vi "RSA306 hkplaying2.vi"() -> ()   [LabVIEW 2016]
doc: "This VI demonstrates a simple procedure for setting up a spectrum analyzer, running an acquisition, and retrieving and plotting the waveform data.\n\nString indicators Binary WF Data and Sgl Float WF Data are initialized to empty strings. Waveform Graph is initialized to 0 for 100000 locations (just an arbitrary number for demonstration purposes).\n\ntkrsa6100 Initialize.vi opens the VISA Resource Name from the information entered by the user. It also presets the instrument by default to the Spectrum measurement. On completion it passes dup VISA Resource Name and error out to the following drivers.\n\nThe next VI to execute is tkrsa6100 Config Frequency.vi. Numeric control Center Freq (MHz)(50) is passed to the VI to set the center frequency to the default 50MHz value. The Set/Read Freq Setting (Set) is not wired since it defaults to SET, which is what is desired in this case. This is the case for all the configuration VI's in the example.\n\nThe next VI to execute is tkrsa6100 Config Spectrum Settings.vi. Enumerated control Spectrum Settings (CENTER FREQUENCY) is passed a Frequency Span constant and numeric control Freq Span (MHz) (40) to set the span to 40MHz.\n\nNext the reference level is set using tkrsa6100 Config RF Input.vi. Enumerated control Input Setting (REFERENCE LEVEL) is passed a Reference Level constant and numeric control Ref Level (dBm)(0) to set the reference level to 0dBm.\n\nNext the acquisition mode is set to single acquisition using tkrsa6100 Config Acquisition.vi. No parameters are passed since the default setting of this VI sets the acquisition mode to single.\n\nA single acquisition is then performed using tkrsa6100 Run Single Acquisition.vi. This VI sends an INIT command followed by a *OPC? Query. When the acquisition is completed the instrument returns a 1 and the next vi executes.\n\nThe binary waveform data is then retrieved by tkrsa6100 Spectrum Msmt Results.vi. The last acquisition data is retrieved by passing constant GET LAST ACQUISITION RESULT to enumerated input Run Acquisition and/or Get Result (RUN ACQUISITION & GET RESULT). The binary data is converted to a comma separated list of single precision floating point numbers by passing constant YES to enumerated input Convert Resp String (NO). The number of display points (total number of data bytes/4) is passed to a Spectral Display property node to scale the x axis of the graph. The binary data string from output Measurement Response String is copied to string indicator Binary WF Data. The converted binary data from output Converted Sgl Float Response String is copied to string indicator Sgl Float WF Data.\n\nSgl Float WF Data is then converted to an array by function Spreadsheet String to Array using a comma as the data separator. The output array is then passed to waveform graph Spectral Display for viewing.\n\nThe VISA Resource Name is closed using tkrsa6100 Close.vi."
panel:
  out "Time to Sample":dbl
  out "Total # of Samples":i32
  in  "Freq Out Cluster":T1={"Start Freq (MHz)"=0.0, "Stop Freq (MHz)"=40.0, "Freq Center"=20000000.0, "Freq Step (KHz)"=49.93757802746566, "Acquisition Time (ms)"=0.2181818181818, "Acquisition Samples"=12218.0, "Time Step (sec)"=1.785740859238828e-08, "Spectrum Length"=0.0234894285714, "Spectrum Offset"=-0.0117447142857}
  in  "Freq Center":dbl
  in  "RSA Control Cluster":T2={"Center Freq (MHz)"=20.0, "Freq Span (MHz)"=40.0, "Ref Level (dBm)"=0.0, "# Points"=enum."801", "Analysis Length (ms)"=0.2, "Trigger Settings\n(TRIGGER SOURCE)"=enum."TRIGGER ON"} {"Analysis Length (ms)" step=1e-09; "Ref Level (dBm)" min=-170.0 max=50.0 step=0.1}
  out "cursor diff":dbl
  out "iteration":i32
  out "# of Pts Between Cursors":dbl
  out "Cursor 1 X":dbl
  out "Cursor 0 X":dbl
  in  "I & Q full":cluster{dbl[], "I or Q Data Array":sgl[]}[](graph)=[{array[11200 elements], "I or Q Data Array"=array[11200 elements]}, {array[11200 elements], "I or Q Data Array"=array[11200 elements]}]
  in  "stop":bool
  in  "beta":dbl format="%0.2f"
  in  "Use windowing":bool
  out "FFT^2 from I&Q":cluster{dbl[], dbl[]}[](graph)
  out "FreqStep":dbl
  out "I & Q  partial":cluster{dbl[], sgl[]}[](graph)
  # "This VI has the setup parameters entered in a sub VI\nThe FFT calculation is done in a loop that allows the # of pts\nto FFT to be selected. Also windowing can be changed.\nWhen happy about the FFT then push the STOP button.\nVersion just h is this VI before the setup sub VI was used.\n4/21/17 Version hj moved the memory full causing for loop out of the \nwhile loop. Also added Trigger source to RSA cluster, so it could be\nset to Trigger Off to allow run without pulseblaster trigger."
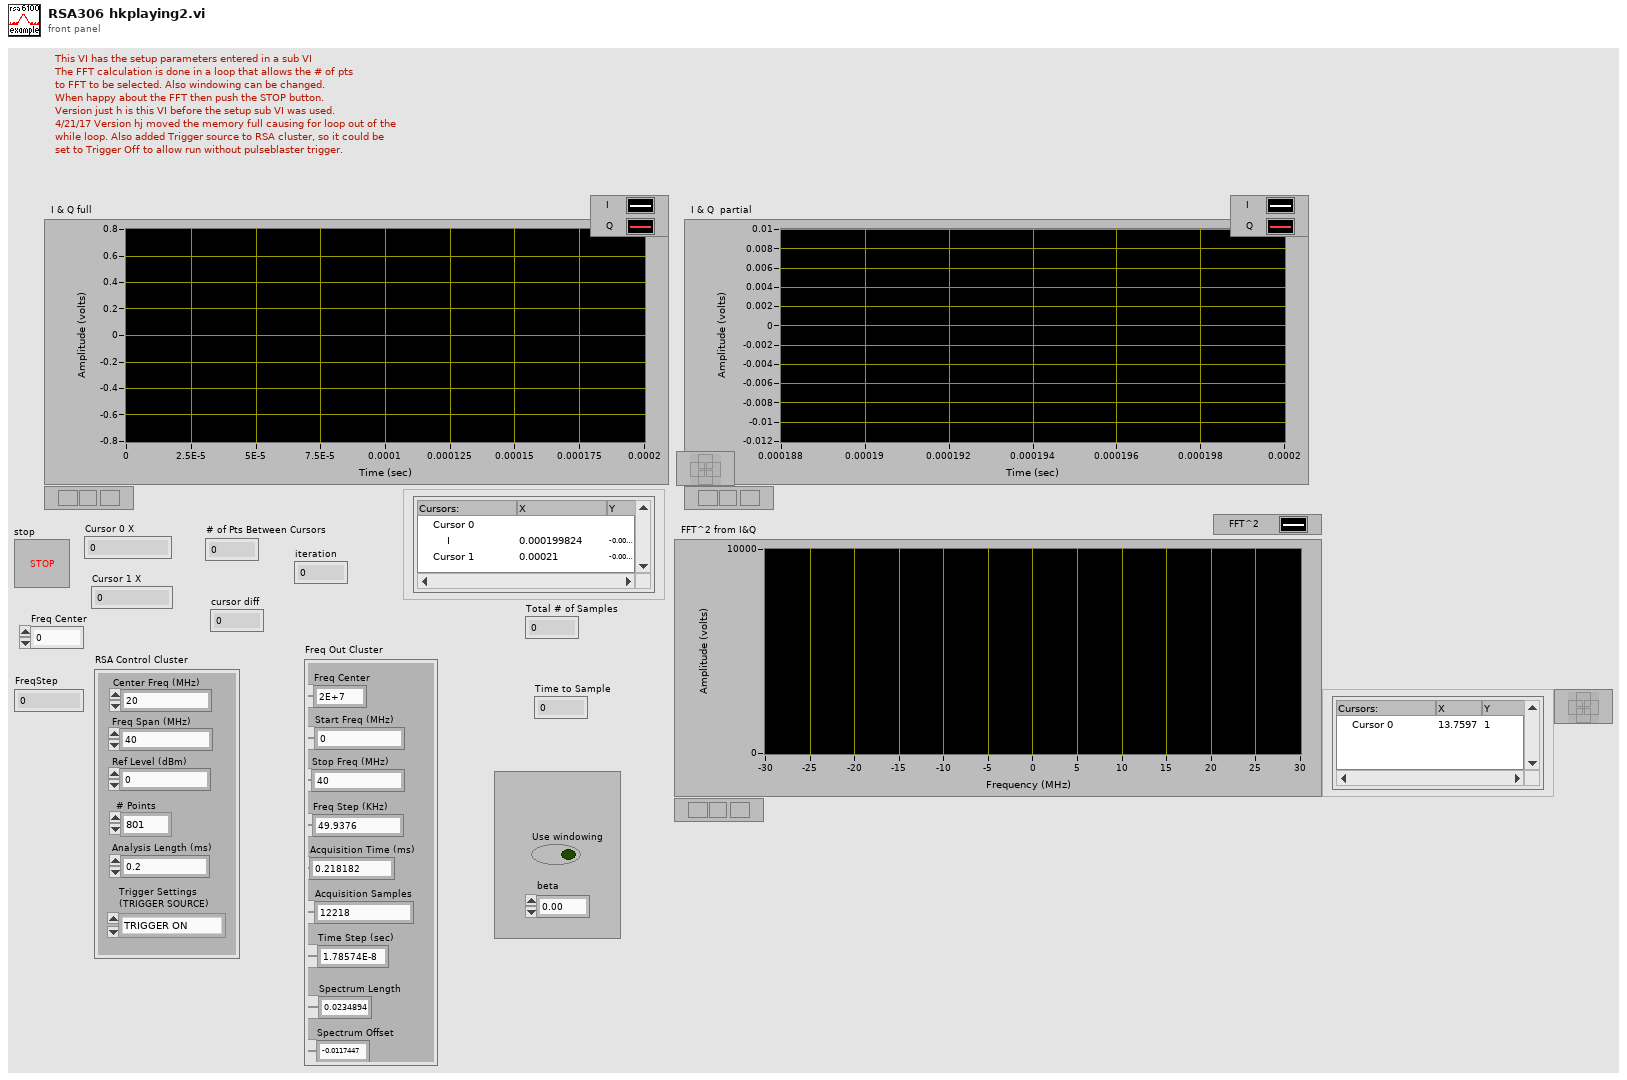
[diagram p1: front panel]
types:
  T1 = cluster{"Start Freq (MHz)":dbl, "Stop Freq (MHz)":dbl, "Freq Center":dbl, "Freq Step (KHz)":dbl, "Acquisition Time (ms)":dbl, "Acquisition Samples":dbl, "Time Step (sec)":dbl, "Spectrum Length":dbl, "Spectrum Offset":dbl}
  T2 = cluster{"Center Freq (MHz)":dbl, "Freq Span (MHz)":dbl, "Ref Level (dBm)":dbl, "# Points":enum16{"801", "2401", "4001", "8001", "10401", "16001", "32001", "64001"}, "Analysis Length (ms)":dbl, "Trigger Settings\n(TRIGGER SOURCE)":enum16{"TRIGGER SOURCE", "TRIGGER ON", "TRIGGER OFF", "TIME DELAY", "TIME POSITION", "TRIGGER EACH SEGMENT ON", "TRIGGER EACH SEGMENT OFF", "TRIGGER HOLDOFF ON", "TRIGGER HOLDOFF OFF", "TRIGGER HOLDOFF TIME", "FRONT EXT  LEVEL", "FRONT EXT IMPEDANCE", "FRONT EXT SLOPE", "REAR EXT SLOPE", "GATED TRIG2 (REAR) LOGIC", "FORCE TRIGGER (SET)"}}
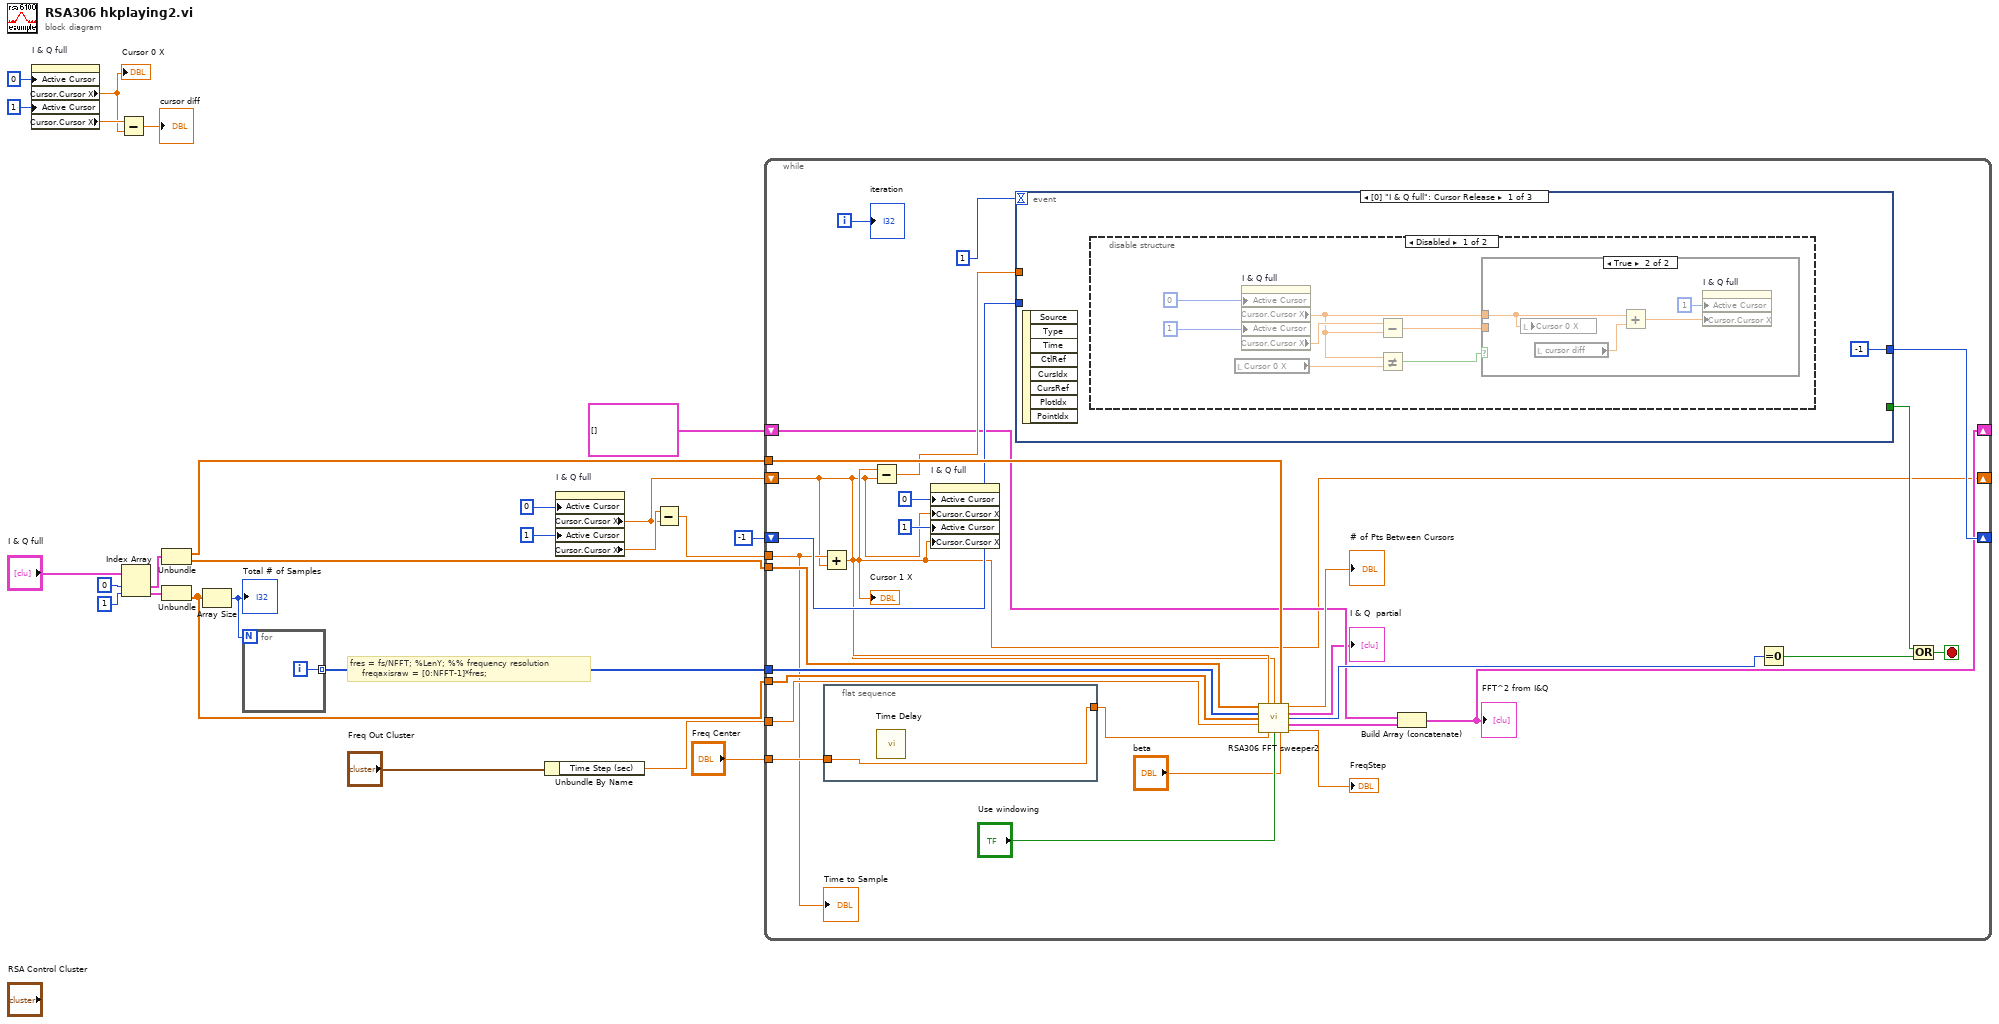
[diagram p0: block diagram]
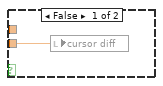
[diagram p2: hidden frame]
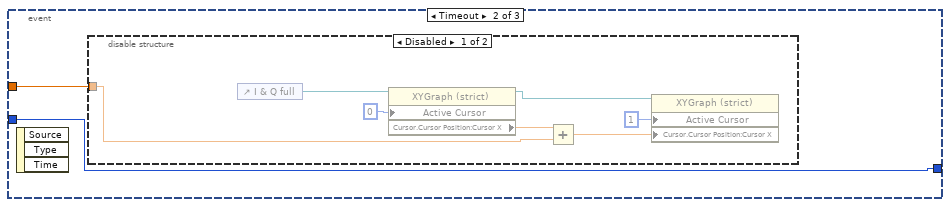
[diagram p4: hidden frame]
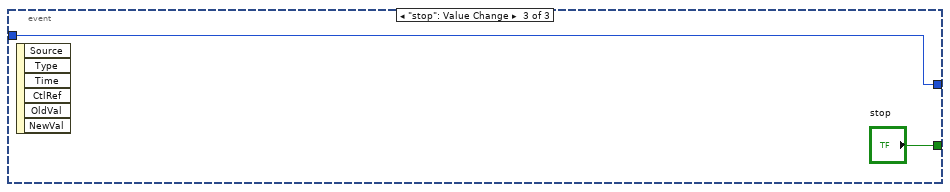
[diagram p6: hidden frame]
diagram:
  # "fres = fs/NFFT; %LenY; %% frequency resolution\n    freqaxisraw = [0:NFFT-1]*fres;"
  n1 = property on="I & Q full" class="XYGraph (strict)"("Active Cursor"=u32 0, "Active Cursor"=u32 1) -> ("Cursor.Cursor X"=w20:dbl, "Cursor.Cursor X"=w22:dbl)  [unwired: 2 in, 2 out]
  "Cursor 0 X" <- w20
  n2 = Subtract(x=w22, y=w20) -> (x-y=→"cursor diff":dbl)
  n3 = Index Array(array="I & Q full", index #1=0 ("index"), index #2=1 ("index")) -> (element #1=w15:cluster{dbl[], "I or Q Data Array":sgl[]}, element #2=w14:cluster{dbl[], "I or Q Data Array":sgl[]})
  n4 = Unbundle(w15) -> (w13:dbl[], "I or Q Data Array"=w12:sgl[])
  n5 = Unbundle(w14) -> ("I or Q Data Array"=w9:sgl[])  [unwired: 1 out]
  n6 = Array Size(array=w9) -> (size(s)=w8:i32)
  "Total # of Samples" <- w8
  n7 = for {
    N: w8 -> [_]
    tunnel: [w26] -> w19 mode=indexing
    i -> [w26]
  }
  n8 = Unbundle By Name("Freq Out Cluster") -> ("Time Step (sec)"=w1:dbl)
  n9 = property on="I & Q full" class="XYGraph (strict)"("Active Cursor"=u32 0, "Active Cursor"=u32 1) -> ("Cursor.Cursor X"=w4:dbl, "Cursor.Cursor X"=w5:dbl)  [unwired: 2 in, 2 out]
  n10 = Subtract(x=w5, y=w4) -> (x-y=w3:dbl)
  n11 = while {
    tunnel: w9 -> [w55]
    tunnel: w12 -> [w54]
    tunnel: "Freq Center" -> [w46]
    tunnel: w13 -> [w52]
    shift-right: [w50] -> _
    shift-left: -1 -> [w51]
    tunnel: w19 -> [w44]
    tunnel: w1 -> [w42]
    shift-right: [w31] -> _
    shift-left: w4 -> [w30]
    tunnel: w3 -> [w33]
    shift-right: [w35] -> _
    shift-left: cluster{dbl[], dbl[]}[] [] -> [w36]
    i -> [w48]
    stop <- w38 stop-if-true
    n12 = Add(x=w33, y=w30) -> (x+y=w31:dbl)
    "Cursor 1 X" <- w31
    n13 = flat-sequence {
      tunnel: w46 -> [w56]
      tunnel: [w56] -> w45
      frame #0 {
        n14 = call "Time Delay"() -> ()  [unwired: 11 in, 1 out]
      }
    }
    n15 = Subtract(x=w31, y=w30) -> (x-y=w49:dbl)
    n16 = property on="I & Q full" class="XYGraph (strict)"("Active Cursor"=u32 0, "Cursor.Cursor X"=w30, "Active Cursor"=u32 1, "Cursor.Cursor X"=w31) -> ()  [unwired: 2 in, 2 out]
    n17 = event shown="[0] \"I & Q full\": Cursor Release" {
      selector: _ -> [_ _ _]
      dyn-events: _ -> [_ _ _]
      timeout: 1 -> [_ _ _]
      tunnel: [_ _ "stop"] -> w39
      tunnel: [-1 w71 w80] -> w50
      tunnel: w51 -> [_ w71 w80]
      tunnel: w49 -> [_ w70 _]
      event "I & Q full": Cursor Release {
        n18 = event-data() -> ()  [unwired: 1 in, 8 out]
        n19 = disable-structure shown="Disabled" {
          frame Disabled {
            n20 = local read "Cursor 0 X"() -> (w62:dbl)
            n21 = property on="I & Q full" class="XYGraph (strict)"("Active Cursor"=u32 0, "Active Cursor"=u32 1) -> ("Cursor.Cursor X"=w59:dbl, "Cursor.Cursor X"=w60:dbl)  [unwired: 2 in, 2 out]
            n22 = Subtract(x=w60, y=w59) -> (x-y=w58:dbl)
            n23 = Not Equal?(x=w59, y=w62) -> (x != y?=w61:bool)
            n24 = case shown="True" w61 {
              tunnel: w59 -> [_ w66]
              tunnel: w58 -> [w65 _]
              frame False {
                n25 = local write "cursor diff"(w65) -> ()
              }
              frame True {
                n26 = local write "Cursor 0 X"(w66) -> ()
                n27 = local read "cursor diff"() -> (w68:dbl)
                n28 = Add(x=w66, y=w68) -> (x+y=w67:dbl)
                n29 = property on="I & Q full" class="XYGraph (strict)"("Active Cursor"=u32 1, "Cursor.Cursor X"=w67) -> ()  [unwired: 2 in, 2 out]
              }
            }
          }
          frame Enabled {
          }
        }
      }
      event Timeout {
        n30 = event-data() -> ()  [unwired: 1 in, 3 out]
        n31 = disable-structure shown="Disabled" {
          disable-tunnel: w70 -> [w72 _]
          frame Disabled {
            n32 = control-ref of="I & Q full"() -> (w73:refnum<vi>)
            n33 = property class="XYGraph (strict)"(reference=w73, "Active Cursor"=u32 0) -> (reference out=w76:refnum<vi>, "Cursor.Cursor Position:Cursor X"=w75:dbl)  [unwired: 1 in, 1 out]
            n34 = Add(x=w75, y=w72) -> (x+y=w74:dbl)
            n35 = property class="XYGraph (strict)"(reference=w76, "Active Cursor"=u32 1, "Cursor.Cursor Position:Cursor X"=w74) -> ()  [unwired: 1 in, 2 out]
          }
          frame Enabled {
          }
        }
      }
      event "stop": Value Change {
        n36 = event-data() -> ()  [unwired: 1 in, 6 out]
      }
    }
    n37 = call "RSA306 FFT sweeper2.vi"("Q Array"=w54, "2nd Cursor X"=w31, "1st Cursor X"=w30, "Time Array"=w52, "1toN Array"=w44, "I Array"=w55, "time step(sec)"=w42, "Freq Center"=w45, "Use windowing"="Use windowing", "beta"="beta") -> ("# of Pts Between cursors"=→"# of Pts Between Cursors":dbl, "I & Q  partial"=→"I & Q  partial":cluster{dbl[], sgl[]}[], "Length out"=w41:i32, "FFT^2 from partial"=w37:cluster{dbl[], dbl[]}, "FreqStep"=→"FreqStep":dbl)  [unwired: 1 in]
    n38 = Build Array (concatenate)(w36, w37) -> (w35:cluster{dbl[], dbl[]}[])
    "FFT^2 from I&Q" <- w35
    n39 = Equal To 0?(x=w41) -> (x = 0?=w40:bool)
    n40 = Or(x=w39, y=w40) -> (x .or. y?=w38:bool)
    "iteration" <- w48
    "Time to Sample" <- w33
  }
